vi "Handle Last Ack Core.vi"(4 "error in (no error)":errorcluster, 6 "Last Ack":refnum<class "Last Ack.lvclass">, 7 "Calling Actor in":refnum<class "Calling Actor.lvclass">) -> (0 "error out":errorcluster, 3 "Calling Actor out":refnum<class "Calling Actor.lvclass">)   [LabVIEW 2019, in "Calling Actor.lvlib" / "Calling Actor.lvclass"]
doc: "(<B>Filename</B>: Actor Framework.lvlib:Actor.lvclass:Handle Last Ack Core.vi)\n\nDefines how the caller actor responds to the Last Ack message from a nested actor. The Last Ack message is the final message a nested actor sends to its caller before it shuts down. The message contains information about the final state of the nested actor.\n\nBy default, this method does nothing except return any error the nested actor sent. A descendant class may override this method to define behavior."
uses:
  Calling Actor.lvclass
  <vilib>/ActorFramework/LastAck/Last Ack.lvclass
  Calling Actor.lvclass/Calling Actor.ctl
  <vilib>/ActorFramework/Actor/Actor.lvclass
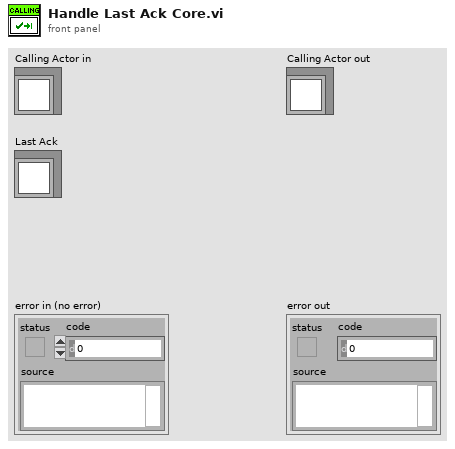
[diagram p1: front panel]
types:
  T1 = map{string, refnum<class "Message Enqueuer.lvclass">}
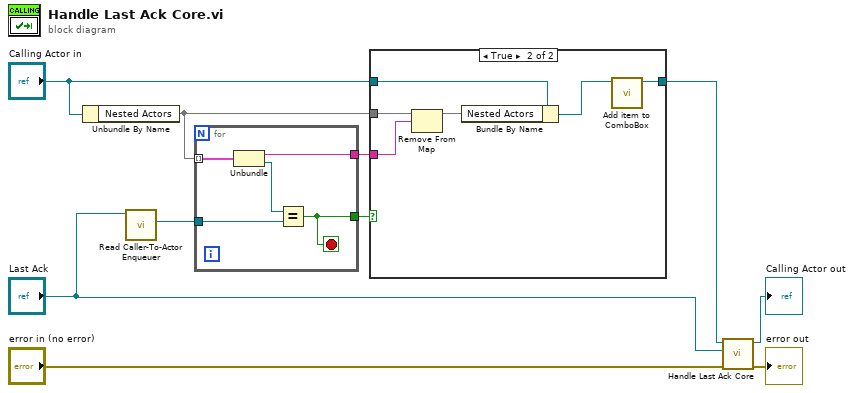
[diagram p0: block diagram]
diagram:
  n1 = Unbundle By Name("Calling Actor in") -> ("Nested Actors"=w5:T1)
  n2 = call <vilib>:"Read Caller-To-Actor Enqueuer.vi"("Last Ack"="Last Ack") -> ("Caller-to-Actor Enqueuer"=w6:refnum<class "Message Enqueuer.lvclass">)  [unwired: 10 in]
  n3 = for {
    tunnel: w5 -> [w15] mode=indexing
    tunnel: w6 -> [w13]
    tunnel: [w12] -> w2
    tunnel: [w11] -> w4
    stop <- w12 stop-if-true
    n4 = Unbundle(w15) -> (w11:string, "Nested Enqueuer"=w14:refnum<class "Message Enqueuer.lvclass">)
    n5 = Equal?(x=w14, y=w13) -> (x = y?=w12:bool)
  }
  n6 = case shown="True" w2 {
    tunnel: w5 -> [_ w22]
    tunnel: w4 -> [_ w21]
    tunnel: "Calling Actor in" -> [w16 w20]
    tunnel: [w16 w17] -> w1
    frame False {
    }
    frame True {
      n7 = Remove From Map(10:w21, 11:w22) -> (3:w19:T1)  [unwired: 2 out]
      n8 = Bundle By Name(cluster=w20, "Nested Actors"=w19) -> (w18:refnum<class "Calling Actor.lvclass">)
      n9 = call "Add item to ComboBox.vi"("Calling Actor in"=w18) -> ("Calling Actor out"=w17:refnum<class "Calling Actor.lvclass">)  [unwired: 9 in, 1 out]
    }
  }
  n10 = call-parent "Handle Last Ack Core.vi"("error in (no error)"="error in (no error)", "Last Ack"="Last Ack", "Actor in"=w1) -> ("error out"=→"error out":errorcluster, "Actor out"=→"Calling Actor out":refnum<class "Calling Actor.lvclass">)  [unwired: 3 in]
